vi "Insert into Object.vi"(5 "JSON to Insert":string, 6 "Item Path":string, 7 "error in (no error)":errorcluster, 9 "Object Offset":i32, 10 "JSON in":string="{}") -> (0 "error out":errorcluster, 1 "Replaced":bool, 3 "<JSON>":string)   [LabVIEW 2013, in "JSONtext.lvlib"]
uses:
  JSONtext.lvlib
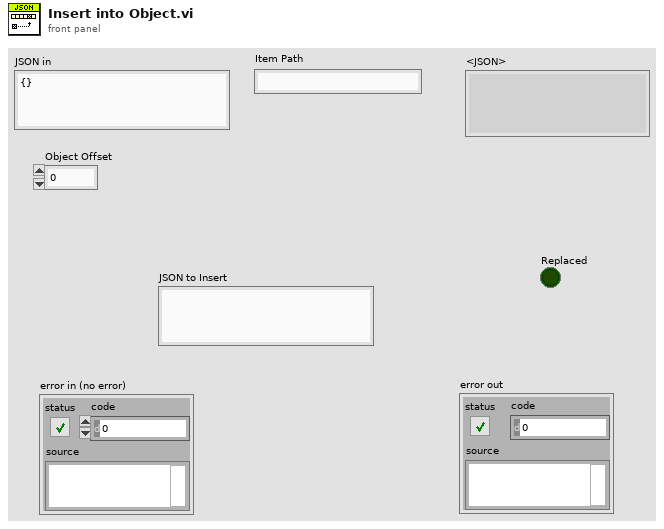
[diagram p1: front panel]
types:
  T1 = typedef "JSONtext.lvlib/Found Items.ctl" = cluster{"Found":bool, "Item offset":i32, "Offset past Item":i32, "Name offset":i32, "Offset past Name":i32, "Empty Object":bool}
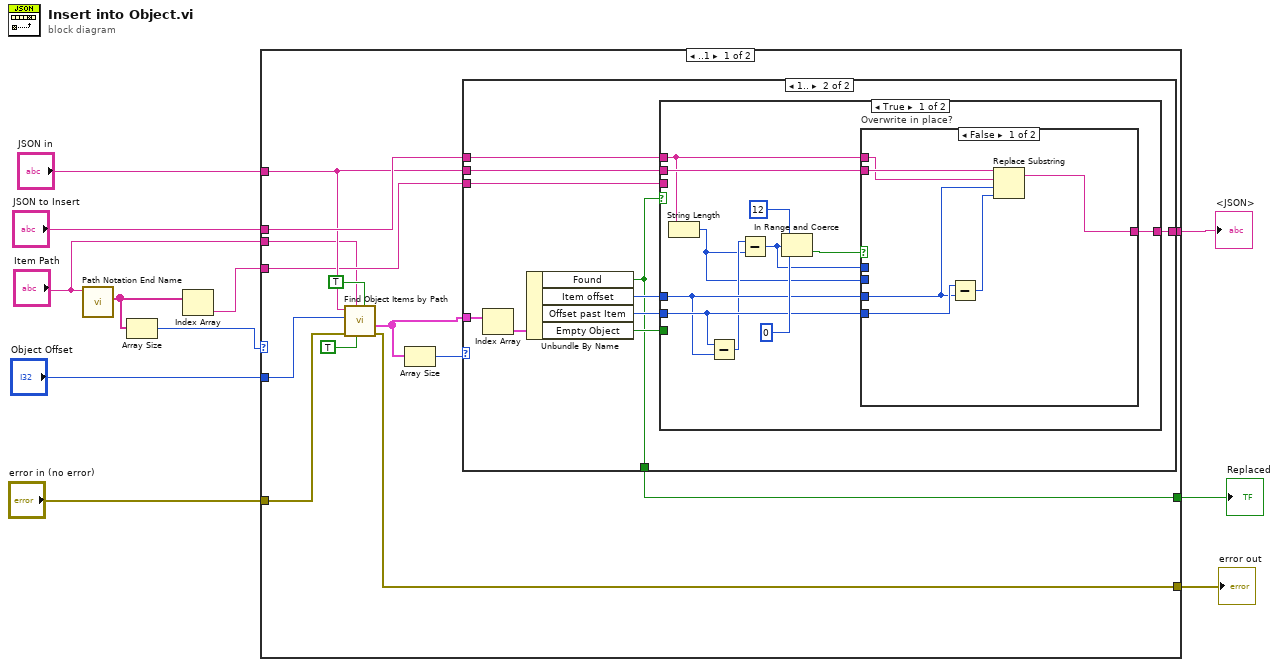
[diagram p0: block diagram]
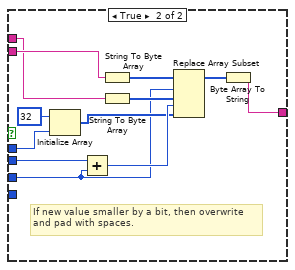
[diagram p3: hidden frame]
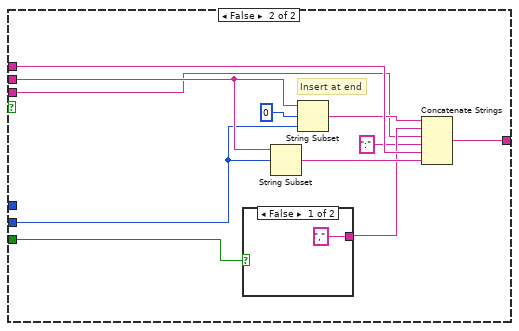
[diagram p4: hidden frame]
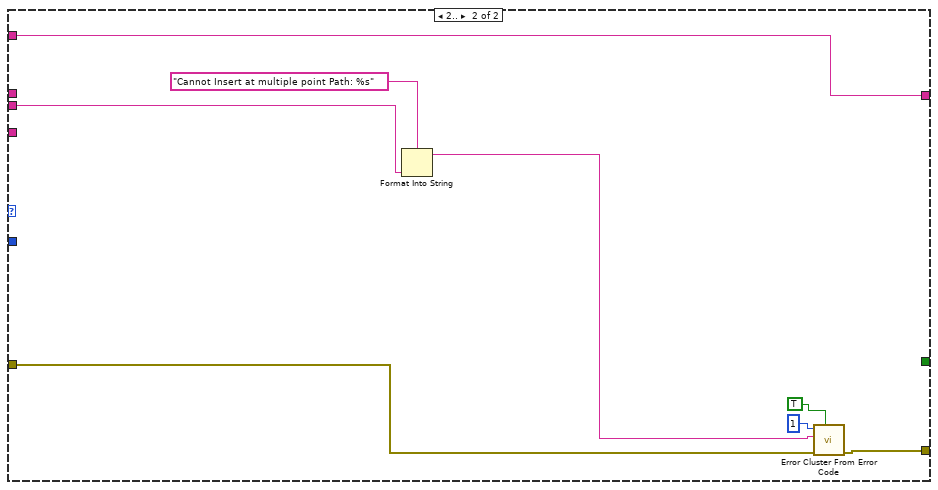
[diagram p6: hidden frame]
diagram:
  n1 = call "Path Notation End Name.vi"("Item Path"="Item Path") -> ("<JSON>End Names"=w2:string[])  [unwired: 10 in]
  n2 = Array Size(array=w2) -> (size(s)=w3:i32)
  n3 = Index Array(array=w2) -> (element=w4:string)  [unwired: 1 in]
  n4 = case shown="..1" w3 {
    tunnel: "JSON to Insert" -> [w24 _]
    tunnel: [w23 w78] -> w10
    tunnel: "JSON in" -> [w22 w78]
    tunnel: "Object Offset" -> [w21 _]
    tunnel: [w17 _] -> w7
    tunnel: "error in (no error)" -> [w16 w79]
    tunnel: [w15 w82] -> w5
    tunnel: w4 -> [w13 _]
    tunnel: "Item Path" -> [w12 w77]
    frame ..1 {
      n5 = call "Find Object Items by Path.vi"("Insertion point if not found"=TRUE, "Only return first found"=TRUE, "Path"=w12, "error in (no error)"=w16, "Object Offset"=w21, "JSON"=w22) -> ("error out"=w15:errorcluster, "Items"=w18:T1[])  [unwired: 4 in]
      n6 = Array Size(array=w18) -> (size(s)=w19:i32)
      n7 = case shown="1.." w19 {
        tunnel: w24 -> [_ w35]
        tunnel: [w25 w34] -> w23
        tunnel: w22 -> [w25 w33]
        tunnel: w13 -> [_ w32]
        tunnel: w18 -> [_ w28]
        tunnel: [_ w26] -> w17
        frame 0, Default {
        }
        frame 1.. {
          n8 = Index Array(array=w28) -> (element=w27:T1)  [unwired: 1 in]
          n9 = Unbundle By Name(w27) -> ("Found"=w26:bool, "Item offset"=w31:i32, "Offset past Item"=w30:i32, "Empty Object"=w29:bool)
          n10 = case shown="True" w26 {
            tunnel: w33 -> [w46 w75]
            tunnel: w35 -> [w44 w74]
            tunnel: [w45 w73] -> w34
            tunnel: w32 -> [_ w65]
            tunnel: w31 -> [w39 _]
            tunnel: w30 -> [w40 w67]
            tunnel: w29 -> [_ w66]
            frame True {
              n11 = String Length(string=w44) -> (length=w36:i32)
              n12 = Subtract(x=w40, y=w39) -> (x-y=w38:i32)
              n13 = Subtract(x=w38, y=w36) -> (x-y=w37:i32)
              n14 = In Range and Coerce(upper limit=12, x=w37, lower limit=0) -> (In Range?=w41:bool)  [unwired: 1 out]
              n15 = case "Overwrite in place?" shown="False" w41 {
                tunnel: w46 -> [w52 w61]
                tunnel: [w50 w59] -> w45
                tunnel: w44 -> [w51 w60]
                tunnel: w39 -> [w48 w54]
                tunnel: w40 -> [w49 _]
                tunnel: w37 -> [_ w58]
                tunnel: w36 -> [_ w53]
                frame False {
                  n16 = Subtract(x=w49, y=w48) -> (x-y=w47:i32)
                  n17 = Replace Substring(2:w47, 3:w48, 4:w51, 5:w52) -> (1:w50:string)  [unwired: 1 out]
                }
                frame True {
                  # "If new value smaller by a bit, then overwrite\nand pad with spaces."
                  n18 = Initialize Array(u8 32, w58) -> (w56:u8[])
                  n19 = Add(x=w53, y=w54) -> (x+y=w57:i32)
                  n20 = String To Byte Array(string=w61) -> (unsigned byte array=w64:u8[])
                  n21 = String To Byte Array(string=w60) -> (unsigned byte array=w63:u8[])
                  n22 = Replace Array Subset(array=w64, new element #1=w63, index #1=w54, new element #2=w56, index #2=w57) -> (w62:u8[])
                  n23 = Byte Array To String(unsigned byte array=w62) -> (string=w59:string)
                }
              }
            }
            frame False {
              # "Insert at end"
              n24 = case shown="False" w66 {
                tunnel: ["," ("string") _] -> w69
                frame False {
                }
                frame True {
                }
              }
              n25 = String Subset(string=w75, offset (0)=w67) -> (substring=w70:string)  [unwired: 1 in]
              n26 = String Subset(string=w75, offset (0)=0 ("Value start in"), length (rest)=w67) -> (substring=w71:string)
              n27 = Concatenate Strings(w71, w69, w65, ":" ("string"), w74, w70) -> (w73:string)
            }
          }
        }
      }
    }
    frame 2.. {
      n28 = Format Into String(format string="Cannot Insert at multiple point Path: %s", w77) -> (resulting string=w80:string)  [unwired: 2 in, 1 out]
      n29 = call <vilib>:"Error Cluster From Error Code.vi"("show call chain? (False)"=TRUE, "error in (no error)"=w79, "error message (\"\")"=w80, "error code (0)"=1) -> ("error out"=w82:errorcluster)  [unwired: 5 in]
    }
  }
  "Replaced" <- w7
  "<JSON>" <- w10
  "error out" <- w5
